vi "Get Base Object Name.vi"(8 "error in (no error)":errorcluster, 11 "Object in":refnum<class>) -> (0 "error out":errorcluster, 3 "Base class name":string)   [LabVIEW 2020, in "Data.lvlib"]
doc: "Get the base class name of a LabVIEW object."
uses:
  Data.lvlib
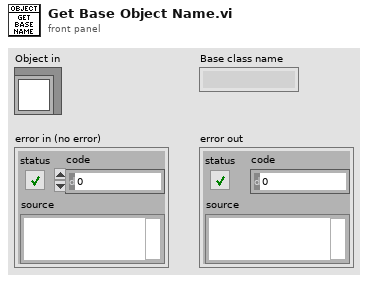
[diagram p1: front panel]
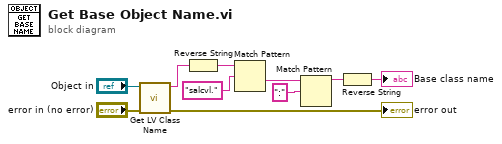
[diagram p0: block diagram]
diagram:
  n1 = call <vilib>:"Get LV Class Name.vi"("error in (no error)"="error in (no error)", "object"="Object in") -> ("error out"=→"error out":errorcluster, "class name"=w4:string)  [unwired: 8 in]
  n2 = Reverse String(1:w4) -> (0:w5:string)
  n3 = Match Pattern(string=w5, regular expression="salcvl.") -> (after substring=w7:string)  [unwired: 1 in, 3 out]
  n4 = Match Pattern(string=w7, regular expression=":") -> (before substring=w9:string)  [unwired: 1 in, 3 out]
  n5 = Reverse String(1:w9) -> (0:→"Base class name":string)
